vi "to negative fixint.vi"(8 "error in":errorcluster, 11 "bytes":u8[](array[numeric]) format="%b") -> (0 "error out":errorcluster, 2 "negative fix int":i8, 3 "remaining bytes":u8[](array[numeric]))   [LabVIEW 2020, in "MessagePack.lvlib" / "MessagePack.lvclass"]
uses:
  MessagePack.lvclass
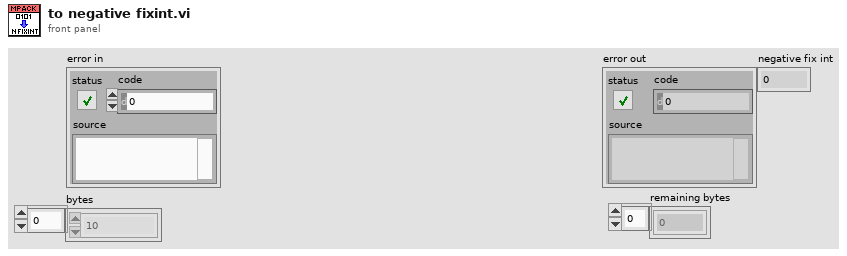
[diagram p1: front panel]
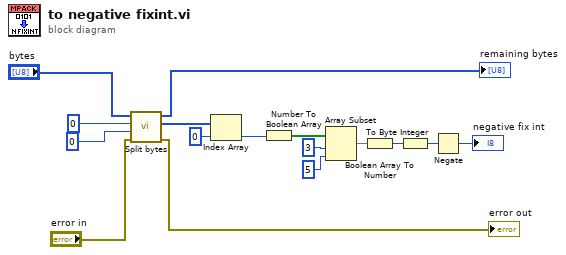
[diagram p0: block diagram]
diagram:
  n1 = call "Split bytes.vi"("error in"="error in", "End index"=0, "Start index"=0, "bytes in"="bytes") -> ("error out"=→"error out":errorcluster, "selected bytes"=w3:u8[], "remaining bytes"=→"remaining bytes":u8[])  [unwired: 4 in, 1 out]
  n2 = Index Array(array=w3, index=0) -> (element=w1:u8)
  n3 = Number To Boolean Array(number=w1) -> (Boolean array=w16:bool[])
  n4 = Array Subset(array=w16, index=3, length=5) -> (w13:bool[])
  n5 = Boolean Array To Number(Boolean array=w13) -> (number=w12:u32)
  n6 = To Byte Integer(number=w12) -> (8bit integer=w11:i8)
  n7 = Negate(x=w11) -> (-x=→"negative fix int":i8)
